vi "DynamicUI.vi"(8 "error in (no error)":errorcluster, 11 "String in":refnum<class "String.lvclass">) -> (0 "error out":errorcluster, 3 "String out":refnum<class "String.lvclass">)   [LabVIEW 2023, in "String.lvclass"]
uses:
  String.lvclass
panel:
  out "String Data":string
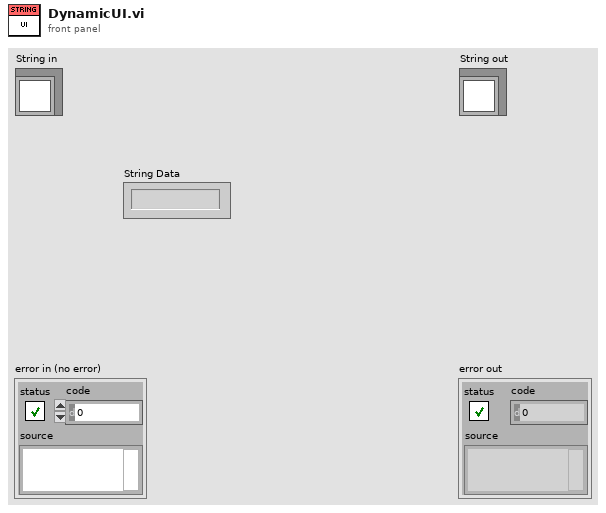
[diagram p1: front panel]
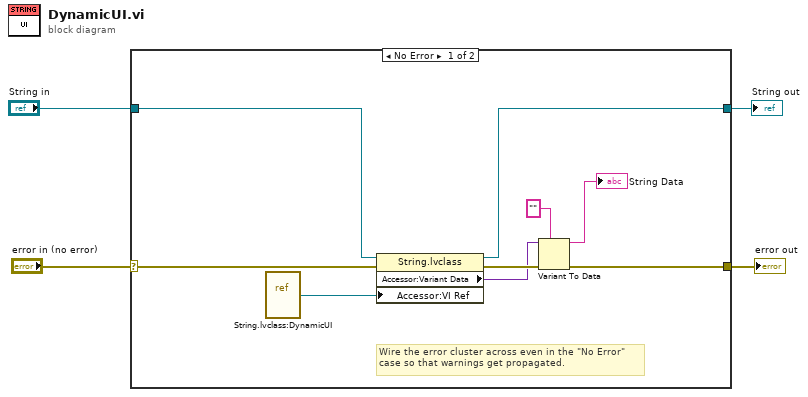
[diagram p0: block diagram]
diagram:
  n1 = case shown="No Error" "error in (no error)" {
    selector: "error in (no error)" -> [w13 w15]
    tunnel: [w9 w15] -> w3
    tunnel: [w10 w14] -> w1
    tunnel: "String in" -> [w11 w14]
    frame No Error {
      # "Wire the error cluster across even in the \"No Error\"\ncase so that warnings get propagated."
      n2 = vi-ref "String.lvclass:DynamicUI.vi"() -> (w5:refnum<vi>)
      n3 = property class="String.lvclass"(reference=w11, error in=w13, "Accessor:VI Ref"=w5) -> (reference out=w10:refnum<class "String.lvclass">, error out=w12:errorcluster, "Accessor:Variant Data"=w8:variant)
      n4 = Variant To Data(error in=w12, type="", Variant=w8) -> (data=→"String Data":string, error out=w9:errorcluster)
    }
    frame Error {
    }
  }
  "error out" <- w3
  "String out" <- w1
